vi "scalar_product.vi"(8 "error in (no error)":errorcluster, 10 "B in":refnum<class "SpaceVector.lvclass">, 11 "A in":refnum<class "SpaceVector.lvclass">) -> (0 "error out":errorcluster, 2 "scalar product":dbl[unit], 3 "A out":refnum<class "SpaceVector.lvclass">)   [LabVIEW 2010, in "SpaceVector.lvclass"]
uses:
  SpaceVector.lvclass
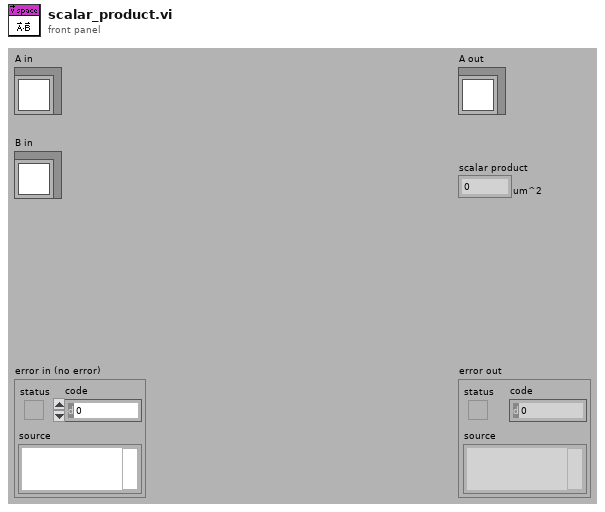
[diagram p1: front panel]
types:
  T1 = typedef "space_vector_array.ctl" = dbl[unit][]
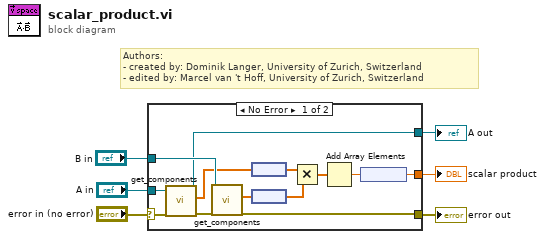
[diagram p0: block diagram]
diagram:
  # "Authors: \n- created by: Dominik Langer, University of Zurich, Switzerland\n- edited by: Marcel van 't Hoff, University of Zurich, Switzerland"
  n1 = case shown="No Error" "error in (no error)" {
    selector: "error in (no error)" -> [w17 w21]
    tunnel: [w15 w21] -> w5
    tunnel: [w14 w20] -> w3
    tunnel: "A in" -> [w19 w20]
    tunnel: "B in" -> [w18 _]
    tunnel: [w7 _] -> w1
    frame No Error {
      n2 = call "get_components.vi"("error in (no error)"=w17, "SpaceVector in"=w19) -> ("error out"=w16:errorcluster, "x/y/z"=w12:T1, "SpaceVector out"=w14:refnum<class "SpaceVector.lvclass">)  [unwired: 4 in, 3 out]
      n3 = call "get_components.vi"("error in (no error)"=w16, "SpaceVector in"=w18) -> ("error out"=w15:errorcluster, "x/y/z"=w10:T1)  [unwired: 4 in, 4 out]
      n4 = node(w12) -> (w11:dbl[])
      n5 = node(w10) -> (w9:dbl[])
      n6 = Multiply(x=w11, y=w9) -> (x*y=w13:dbl[])
      n7 = Add Array Elements(numeric array=w13) -> (sum=w8:dbl)
      n8 = node(w8) -> (w7:dbl[unit])
    }
    frame Error {
    }
  }
  "error out" <- w5
  "A out" <- w3
  "scalar product" <- w1
